vi "New.vi"(5 "Coordinates in":T1, 6 "Size in":dbl, 7 "Mass in":dbl, 9 "color in":u32(colorbox), 10 "Period (ms) in":dbl) -> (3 "Flying Saucer out":refnum<class "Flying Saucer.lvclass">)   [LabVIEW 2021, in "Flying Saucer.lvclass"]
doc: "MIT Licence\nCopyright (c) 2024 David Grollier"
uses:
  Flying Saucer.lvclass
  C:/Users/David/Documents/GameSoccerSpace/Source/Game Componants/Game Board Component/Movable/Movable.lvclass
  C:/Users/David/Documents/GameSoccerSpace/Source/Game Componants/Game Board Component/Game Board Component.lvclass
  C:/Users/David/Documents/GameSoccerSpace/Source/Game Componants/Game Componants.lvclass
  Type Def/Coordinates.ctl
  Type Def/Velocity.ctl
  Movable.lvclass/Movable.ctl
  Game Board Component.lvclass/Game Board Component.ctl
  Game Componants.lvclass/Game Componants.ctl
  Flying Saucer.lvclass/Flying Saucer.ctl
  Movable.lvclass
  Game Board Component.lvclass
  Game Componants.lvclass
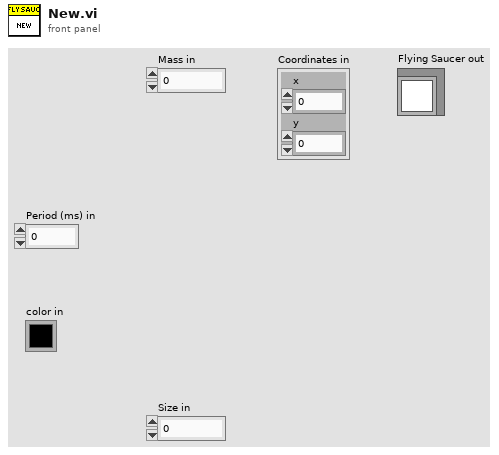
[diagram p1: front panel]
types:
  T1 = typedef "Coordinates.ctl" = cluster{"x":dbl, "y":dbl}
  T2 = typedef "Velocity.ctl" = cluster{"Vx":dbl, "Vy":dbl}
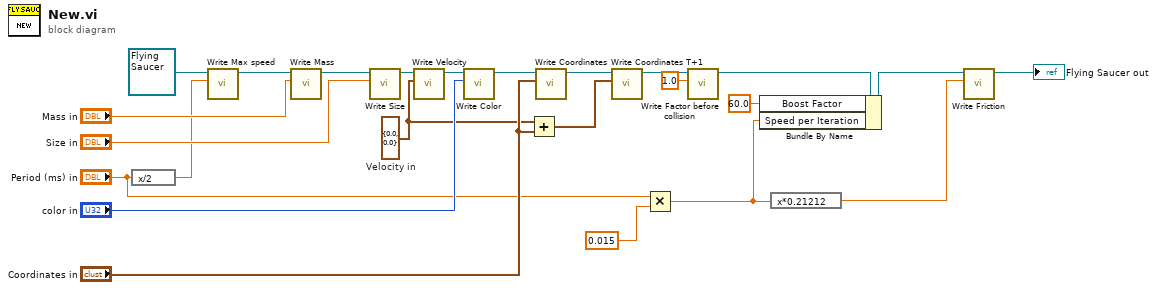
[diagram p0: block diagram]
diagram:
  w9 = T2 {"Vx"=0.0, "Vy"=0.0}  # Velocity in
  n1 = expression code="x/2"("Period (ms) in") -> (w5:dbl)
  n2 = call "Write Max speed.vi"("Max speed"=w5, "Movable in"=refnum<class "Flying Saucer.lvclass"> refnum ("Ball in")) -> ("Movable out"=w11:refnum<class "Flying Saucer.lvclass">)  [unwired: 9 in]
  n3 = call "Write Mass.vi"("Mass"="Mass in", "Movable in"=w11) -> ("Movable out"=w23:refnum<class "Flying Saucer.lvclass">)  [unwired: 9 in]
  n4 = call "Write Size.vi"("Size"="Size in", "Movable in"=w23) -> ("Movable out"=w22:refnum<class "Flying Saucer.lvclass">)  [unwired: 9 in]
  n5 = call "Write Velocity.vi"("Velocity"=w9, "Movable in"=w22) -> ("Movable out"=w19:refnum<class "Flying Saucer.lvclass">)  [unwired: 9 in]
  n6 = call "Write Color.vi"("color"="color in", "Game Board Component in"=w19) -> ("Game Board Component out"=w17:refnum<class "Flying Saucer.lvclass">)  [unwired: 9 in]
  n7 = Add(x=w9, y="Coordinates in") -> (x+y=w10:T2)
  n8 = call "Write Coordinates.vi"("Coordinates"="Coordinates in", "Game Componants in"=w17) -> ("Game Componants out"=w16:refnum<class "Flying Saucer.lvclass">)  [unwired: 9 in]
  n9 = call "Write Coordinates T+1.vi"("Coordinates"=w10, "Movable in"=w16) -> ("Movable out"=w13:refnum<class "Flying Saucer.lvclass">)  [unwired: 9 in]
  n10 = Multiply(x="Period (ms) in", y=0.015) -> (x*y=w3:dbl)
  n11 = call "Write Factor before collision.vi"("Factor before collision"=1.0, "Movable in"=w13) -> ("Movable out"=w15:refnum<class "Flying Saucer.lvclass">)  [unwired: 9 in]
  n12 = Bundle By Name(cluster=w15, "Boost Factor"=60.0 ("Speed per iteration"), "Speed per Iteration"=w3) -> (w8:refnum<class "Flying Saucer.lvclass">)
  n13 = expression code="x*0.21212"(w3) -> (w1:dbl)
  n14 = call "Write Friction.vi"("Friction"=w1, "Movable in"=w8) -> ("Movable out"=→"Flying Saucer out":refnum<class "Flying Saucer.lvclass">)  [unwired: 9 in]
